vi "Set Constant Variables.vi"   [LabVIEW 2012]
uses:
  Robot Global Data.vi
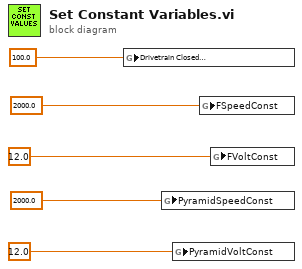
[diagram p0: block diagram]
diagram:
  n1 = global write "Robot Global Data.vi" "Drivetrain Closed\nLoop Max"(100.0 ("Drivetrain Closed\nLoop Max")) -> ()
  n2 = global write "Robot Global Data.vi" "PyramidSpeedConst"(2000.0 ("FSpeedConst")) -> ()
  n3 = global write "Robot Global Data.vi" "PyramidVoltConst"(12.0 ("FVoltConst")) -> ()
  n4 = global write "Robot Global Data.vi" "FSpeedConst"(2000.0 ("FSpeedConst")) -> ()
  n5 = global write "Robot Global Data.vi" "FVoltConst"(12.0 ("FVoltConst")) -> ()
